vi "angle and distance.vi"() -> ()   [LabVIEW 2017]
panel:
  out "Array 2":dbl[](array[numeric])
  out "Array":dbl[](array[numeric])
  out "x*y":dbl
  out "1/x":dbl
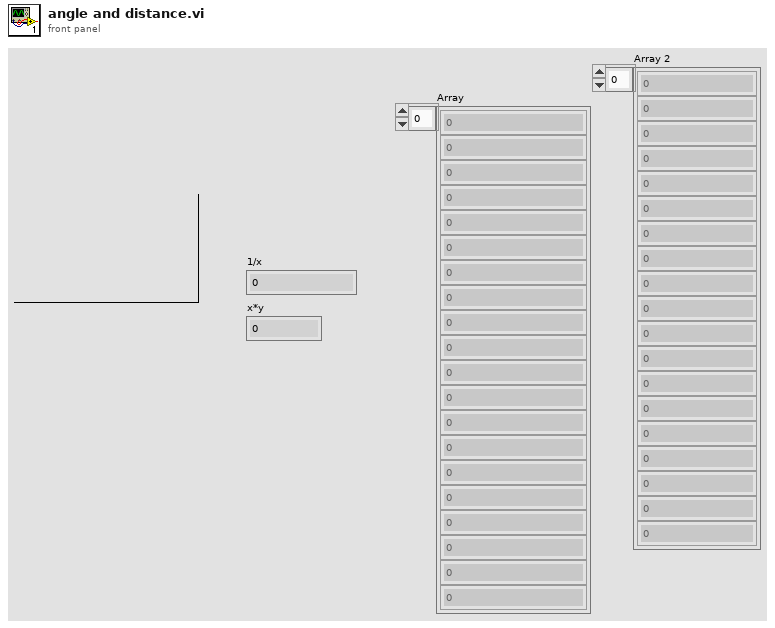
[diagram p1: front panel]
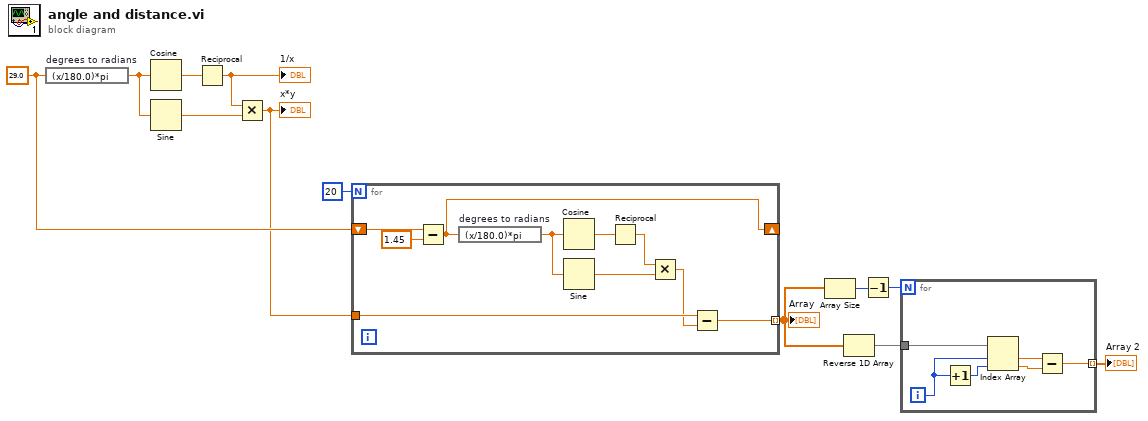
[diagram p0: block diagram]
diagram:
  w7 = 29.0 ("x")
  n1 = expression code="(x/180.0)*pi" "degrees to radians"(w7) -> (w10:dbl)
  n2 = Cosine(x=w10) -> (cos(x)=w12:dbl)
  n3 = Sine(x=w10) -> (sin(x)=w9:dbl)
  n4 = Reciprocal(x=w12) -> (1/x=w11:dbl)
  "1/x" <- w11
  n5 = Multiply(x=w11, y=w9) -> (x*y=w6:dbl)
  "x*y" <- w6
  n6 = for {
    N: 20 -> [_]
    shift-right: [w14] -> _
    shift-left: w7 -> [w22]
    tunnel: w6 -> [w16]
    tunnel: [w13] -> w4 mode=indexing
    n7 = Subtract(x=w22, y=1.45) -> (x-y=w14:dbl)
    n8 = expression code="(x/180.0)*pi" "degrees to radians"(w14) -> (w18:dbl)
    n9 = Cosine(x=w18) -> (cos(x)=w20:dbl)
    n10 = Sine(x=w18) -> (sin(x)=w17:dbl)
    n11 = Reciprocal(x=w20) -> (1/x=w19:dbl)
    n12 = Multiply(x=w19, y=w17) -> (x*y=w15:dbl)
    n13 = Subtract(x=w16, y=w15) -> (x-y=w13:dbl)
  }
  "Array" <- w4
  n14 = Array Size(array=w4) -> (size(s)=w2:i32)
  n15 = Reverse 1D Array(array=w4) -> (reversed array=w5:dbl[])
  n16 = Decrement(x=w2) -> (x-1=w3:i32)
  n17 = for {
    N: w3 -> [_]
    tunnel: w5 -> [w28]
    tunnel: [w23] -> w1 mode=indexing
    i -> [w26]
    n18 = Increment(x=w26) -> (x+1=w27:i32)
    n19 = Index Array(array=w28, index #1=w26, index #2=w27) -> (element #1=w25:dbl, element #2=w24:dbl)
    n20 = Subtract(x=w25, y=w24) -> (x-y=w23:dbl)
  }
  "Array 2" <- w1
